vi "Create Welcome Item.vi"(8 "error in (no error)":errorcluster, 11 "Welcome in":refnum<class "Welcome.lvclass">) -> (0 "error out":errorcluster, 3 "Welcome out":refnum<class "Welcome.lvclass">)   [LabVIEW 2015, in "Item Actor.lvlib" / "Welcome.lvclass"]
uses:
  Welcome.lvclass
  <vilib>/picture/picture.llb/imagedata.ctl
  Generic Item/Generic Item.lvclass/Generic Item.ctl
  Generic Item/Write Weight.vi
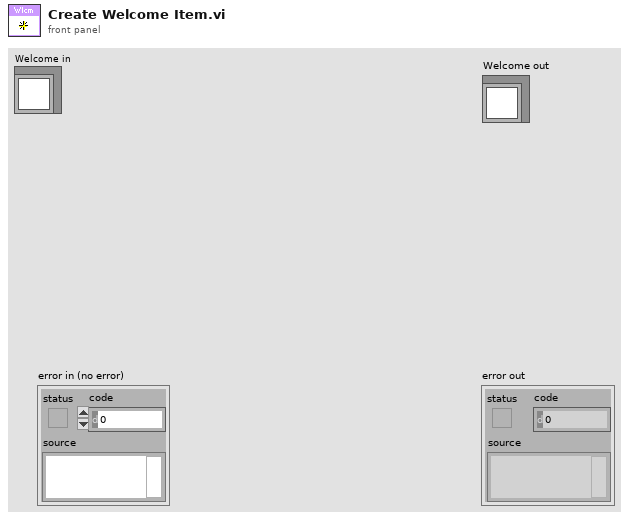
[diagram p1: front panel]
types:
  T1 = typedef "imagedata.ctl" = cluster{"image type":i32, "image depth":i32, "image":u8[], "mask":u8[], "colors":u32[], "Rectangle":cluster{"left":i16, "top":i16, "right":i16, "bottom":i16}}
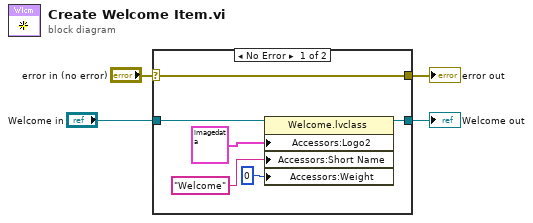
[diagram p0: block diagram]
diagram:
  n1 = case shown="No Error" "error in (no error)" {
    selector: "error in (no error)" -> [w10 w12]
    tunnel: [w10 w12] -> w3
    tunnel: [w8 w11] -> w1
    tunnel: "Welcome in" -> [w9 w11]
    frame No Error {
      n2 = property class="Welcome.lvclass"(reference=w9, "Accessors:Logo2"=T1 {"image type"=0, "image depth"=32, "image"=array[16384 elements], "mask"=[0, 255, 255, 255, 255, 255, 255, 0, 3, 255, 255, 255, 255, 255, 255, 192, 7, 255, 255, 255, 255, 255, 255, 224, 31, 255, 255, 255, 255, 255, 255, 248, 31, 255, 255, 255, 255, 255, 255, 248, 63, 255, 255, 255, 255, 255, 255, 252, 127, 255, 255, 255, 255, 255, 255, 254, 127, 255, 255, 255, 255, 255, 255, 254, 255, 255, 255, 255, 255, 255, 255, 255, 255, 255, 255, 255, 255, 255, 255, 255, 255, 255, 255, 255, 255, 255, 255, 255, 255, 255, 255, 255, 255, 255, 255, 255, 255, 255, 255, 255, 192, 0, 0, 127, 255, 255, 255, 255, 192, 0, 0, 127, 255, 255, 255, 255, 128, 0, 0, 127, 255, 255, 255, 255, 128, 0, 0, 127, 255, 255, 255, 255, 128, 0, 0, 127, 255, 255, 255, 255, 0, 0, 0, 127, 255, 255, 255, 255, 1, 255, 255, 255, 255, 255, 255, 255, 3, 255, 255, 255, 255, 255, 255, 254, 3, 255, 255, 255, 255, 255, 255, 254, 3, 255, 255, 255, 255, 255, 255, 254, 7, 255, 255, 255, 255, 255, 255, 252, 7, 240, 31, 255, 255, 255, 255, 252, 7, 240, 31, 255, 255, 255, 255, 252, 15, 240, 31, 255, 255, 255, 255, 248, 15, 240, 31, 255, 254, 0, 63, 248, 15, 240, 31, 255, 254, 0, 31, 248, 31, 240, 31, 255, 254, 0, 31, 248, 31, 240, 31, 255, 254, 0, 15, 240, 31, 240, 31, 255, 254, 0, 15, 240, 63, 240, 31, 255, 254, 0, 15, 240, 63, 240, 31, 255, 255, 252, 7, 224, 63, 240, 31, 255, 255, 254, 7, 224, 63, 240, 31, 255, 255, 254, 3, 224, 127, 240, 31, 255, 255, 255, 3, 192, 127, 240, 31, 255, 255, 255, 3, 192, 127, 240, 31, 255, 255, 255, 1, 192, 255, 240, 31, 255, 255, 255, 129, 128, 255, 240, 31, 255, 255, 255, 128, 128, 255, 240, 31, 255, 255, 255, 192, 129, 255, 240, 31, 255, 255, 255, 192, 1, 255, 240, 31, 255, 255, 255, 192, 1, 255, 240, 31, 255, 255, 255, 224, 3, 255, 240, 31, 255, 255, 255, 224, 3, 255, 240, 31, 255, 255, 255, 240, 3, 255, 240, 31, 255, 255, 255, 240, 7, 255, 240, 31, 255, 255, 255, 240, 7, 255, 240, 31, 255, 255, 255, 248, 7, 255, 240, 31, 255, 255, 255, 248, 15, 255, 240, 31, 255, 255, 255, 252, 15, 255, 240, 31, 255, 255, 255, 255, 255, 255, 255, 255, 255, 255, 255, 255, 255, 255, 255, 255, 255, 255, 255, 255, 255, 255, 255, 255, 255, 255, 255, 255, 255, 255, 255, 255, 255, 127, 255, 255, 255, 255, 255, 255, 254, 127, 255, 255, 255, 255, 255, 255, 254, 63, 255, 255, 255, 255, 255, 255, 252, 31, 255, 255, 255, 255, 255, 255, 248, 31, 255, 255, 255, 255, 255, 255, 248, 7, 255, 255, 255, 255, 255, 255, 224, 3, 255, 255, 255, 255, 255, 255, 192, 0, 255, 255, 255, 255, 255, 255, 0], "colors"=[], "Rectangle"={"left"=0, "top"=0, "right"=64, "bottom"=64}} ("image data"), "Accessors:Short Name"="Welcome" ("Short Name"), "Accessors:Weight"=0 ("Weight")) -> (reference out=w8:refnum<class "Welcome.lvclass">)  [unwired: 1 in, 1 out]
    }
    frame Error {
    }
  }
  "error out" <- w3
  "Welcome out" <- w1
